vi "DCA Adjust Limit with Waveform Data.vi"(7 "Limit":T1, 8 "error in (no error)":errorcluster, 9 "Data Waveform":waveform(dbl)={"t0"=timestamp(0 s since 1904-01-01), "dt"=0.0, "Y"=[]}) -> (0 "error out":errorcluster, 5 "Modified Limit":T1)   [LabVIEW 2011]
uses:
  TypeDefs/DCA Limit.ctl
  TypeDefs/DCA Limit Quantity.ctl
  TypeDefs/DCA Limit Comparison.ctl
  TypeDefs/DCA Limit Operation.ctl
  Test Referential Limit.ctl
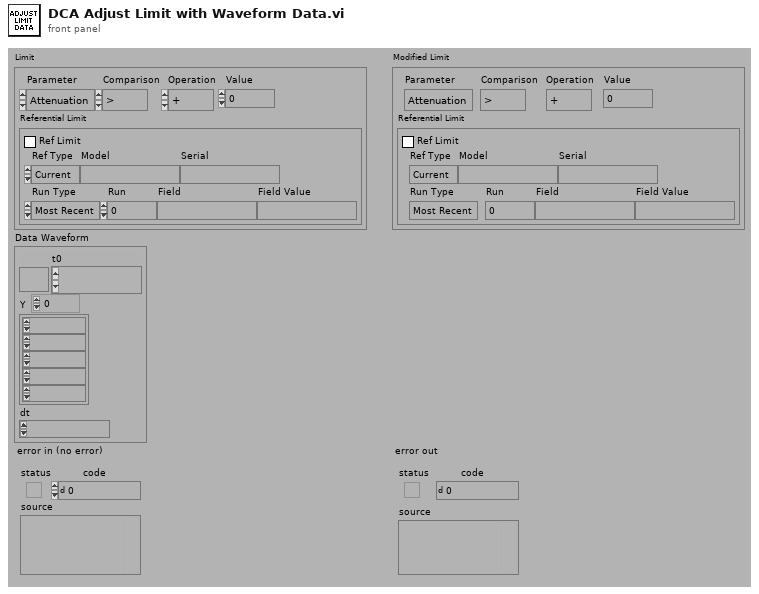
[diagram p1: front panel]
types:
  T1 = typedef "DCA Limit.ctl" = cluster{"Parameter":T2, "Comparison":T3, "Operation":T4, "Value":dbl, "Referential Limit":T5}
  T2 = typedef "DCA Limit Quantity.ctl" = enum16{"Attenuation", "Zin", "Zout", "R1", "R2", "R3", "Rab", "Rac", "Rbc"}
  T3 = typedef "DCA Limit Comparison.ctl" = enum16{">", ">=", "<", "<="}
  T4 = typedef "DCA Limit Operation.ctl" = enum16{"+", "-"}
  T5 = typedef "Test Referential Limit.ctl" = cluster{"Ref Limit":bool, "Ref Type":enum16{"Current", "Specify"}, "Model":string, "Serial":string, "Run Type":enum16{"Most Recent", "Run #", "Match Field"}, "Run":i32, "Field":string, "Field Value":string}
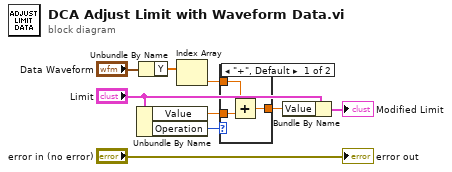
[diagram p0: block diagram]
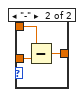
[diagram p2: hidden frame]
diagram:
  n1 = Unbundle By Name("Limit") -> ("Value"=w3:dbl, "Operation"=w1:T4)
  n2 = Unbundle By Name("Data Waveform") -> ("Y"=w5:dbl[])
  n3 = Index Array(array=w5) -> (element=w4:dbl)  [unwired: 1 in]
  n4 = case shown="\"+\", Default" w1 {
    tunnel: w4 -> [w12 w15]
    tunnel: w3 -> [w11 w14]
    tunnel: [w10 w13] -> w2
    frame "+", Default {
      n5 = Add(x=w12, y=w11) -> (x+y=w10:dbl)
    }
    frame "-" {
      n6 = Subtract(x=w15, y=w14) -> (x-y=w13:dbl)
    }
  }
  n7 = Bundle By Name(cluster="Limit", "Value"=w2) -> (→"Modified Limit":T1)
  "error out" <- "error in (no error)"
